vi "HORNSCAN_PERFORMANCE_40KHZ.vi"() -> ()   [LabVIEW 2017]
panel:
  out "Test Result":picture
  out "XY Graph":cluster{dbl, u32}[](graph)
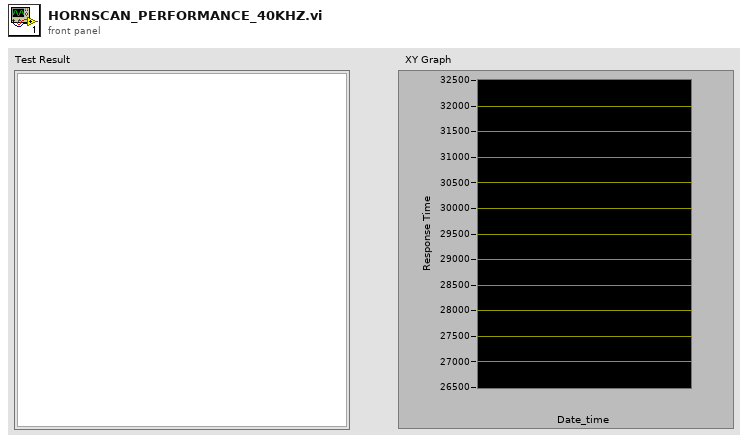
[diagram p1: front panel]
types:
  T1 = enum16{"open", "replace", "create", "open or create", "replace or create", "replace or create with confirmation"}
  T2 = cluster{"[0]":string, "[1]":string, "[2]":string, "[3]":string, "[4]":string, "[5]":string, "[6]":string, "[7]":string, "[8]":string}
  T3 = cluster{"Iterations":u64, "DelayBetweenIterations":u32, "Timeout":u32, "MessageID":i32, "MessageLength":i32, "ResponseID":i32, "Timestamp":string, "TestSuite":string, "ReportPath":path, "FWVersionPath":path}
  T4 = cluster{"Socket_IP_Address":string, "Socket_Port_Number":u16, "Global_ReportPath":path}
  T5 = typedef "imagedata.ctl" = cluster{"image type":i32, "image depth":i32, "image":u8[], "mask":u8[], "colors":u32[], "Rectangle":cluster{"left":i16, "top":i16, "right":i16, "bottom":i16}}
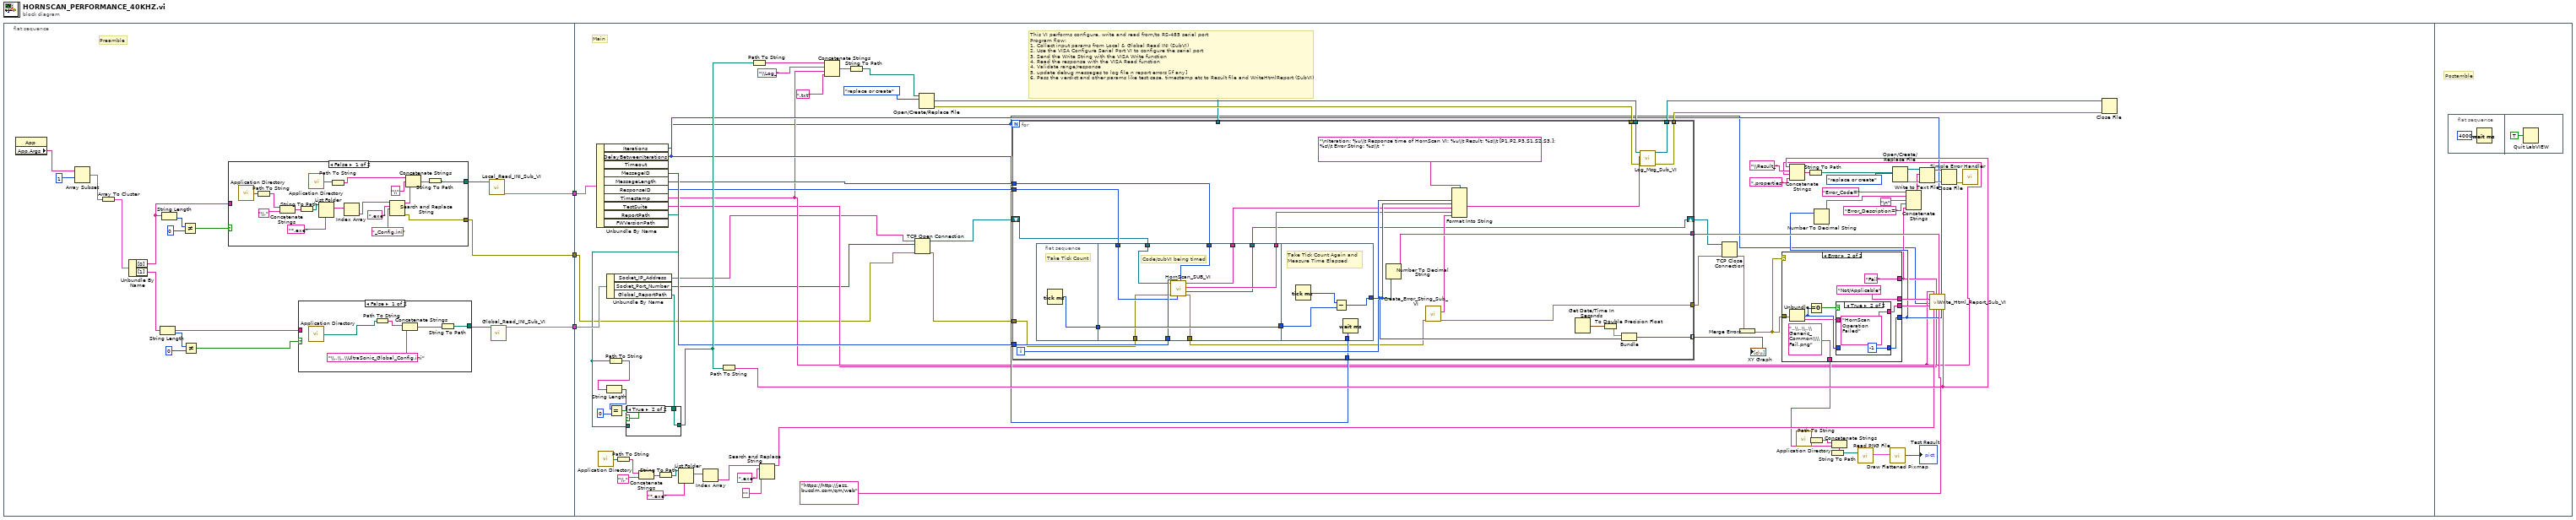
[diagram p0: block diagram]
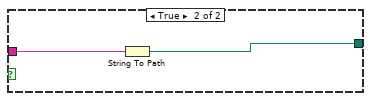
[diagram p2: hidden frame]
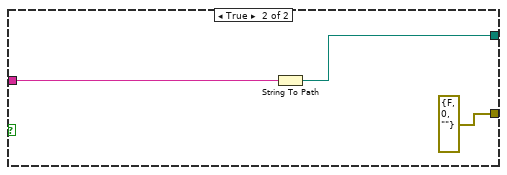
[diagram p3: hidden frame]
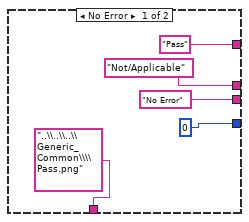
[diagram p5: hidden frame]
diagram:
  n1 = flat-sequence {
    tunnel: [w6] -> w3
    tunnel: [w5] -> w2
    tunnel: [w4] -> w1
    tunnel: w3 -> [w55]
    tunnel: w2 -> [w67]
    tunnel: w1 -> [w65]
    frame #0 {
      # "Preamble"
      n2 = property class="App"() -> ("App.Args"=w8:string[])  [unwired: 2 in, 2 out]
      n3 = Array Subset "Array Subset"(array=w8, index=1) -> (w9:string[])  [unwired: 1 in]
      n4 = Array To Cluster(array=w9) -> (cluster=w10:T2)
      n5 = Unbundle By Name "Unbundle By Name"(w10) -> ("[0]"=w14:string, "[1]"=w17:string)
      n6 = String Length(string=w17) -> (length=w18:i32)
      n7 = String Length(string=w14) -> (length=w11:i32)
      n8 = Not Equal?(x=w11, y=0) -> (x != y?=w13:bool)
      n9 = Not Equal?(x=w18, y=0) -> (x != y?=w16:bool)
      n10 = case shown="False" w13 {
        tunnel: w14 -> [_ w47]
        tunnel: [w29 w46] -> w19
        tunnel: [w28 errorcluster {"status"=FALSE, "code"=0, "source"=""} ("error out")] -> w6
        frame False {
          n11 = call <vilib>:"Application Directory.vi"() -> ("Application Directory"=w35:path)
          n12 = Path To String(path=w35) -> (string=w34:string)
          n13 = Concatenate Strings(w34, "\\." ("string")) -> (w32:string)
          n14 = String To Path(string=w32) -> (path=w37:path)
          n15 = call <vilib>:"Application Directory.vi"() -> ("Application Directory"=w44:path)
          n16 = List Folder(path=w37, pattern="*.exe") -> (filenames=w31:string[])  [unwired: 2 in, 3 out]
          n17 = Path To String(path=w44) -> (string=w39:string)
          n18 = Index Array(array=w31) -> (element=w30:string)  [unwired: 1 in]
          n19 = Search and Replace String(input string=w30, search string=".exe", replace string="_Config.ini" ("replace string (\"\")")) -> (result string=w41:string, error out=w28:errorcluster)  [unwired: 5 in, 2 out]
          n20 = Concatenate Strings(w39, "\\" ("string"), w41) -> (w38:string)
          n21 = String To Path(string=w38) -> (path=w29:path)
        }
        frame True {
          n22 = String To Path(string=w47) -> (path=w46:path)
        }
      }
      n23 = case shown="False" w16 {
        tunnel: [w22 w27] -> w20
        tunnel: w17 -> [_ w26]
        frame False {
          n24 = call <vilib>:"Application Directory.vi"() -> ("Application Directory"=w21:path)
          n25 = Path To String(path=w21) -> (string=w25:string)
          n26 = Concatenate Strings(w25, "\\..\\..\\UltraSonic_Global_Config.ini" ("string")) -> (w23:string)
          n27 = String To Path(string=w23) -> (path=w22:path)
        }
        frame True {
          n28 = String To Path(string=w26) -> (path=w27:path)
        }
      }
      n29 = call "Local_Read_INI_Sub_VI.vi"("Config File Path"=w19) -> ("output cluster"=w4:T3)  [unwired: 10 in]
      n30 = call "Global_Read_INI_Sub_VI.vi"("Config File Path"=w20) -> ("output cluster"=w5:T4)  [unwired: 14 in]
    }
    frame #1 {
      # "This VI performs configure, write and read from/to RS-485 serial port\nProgram flow:\n1. Collect input params from Local & Global Read INI (SubVI)\n2. Use the VISA Configure Serial Port VI to configure the serial port\n3. Send the Write String with the VISA Write function\n4. Read the response with the VISA Read function\n4. Validate range/response\n5. update debug messages to log file n report errors [if any]\n6. Pass the verdict and other params like test case, timestamp etc to Result file and WriteHtmlReport (SubVI)"
      # "Main"
      n31 = Unbundle By Name(w65) -> ("Iterations"=w57:u64, "DelayBetweenIterations"=w61:u32, "MessageID"=w64:i32, "MessageLength"=w63:i32, "ResponseID"=w62:i32, "Timestamp"=w59:string, "TestSuite"=w58:string, "ReportPath"=w56:path)  [unwired: 2 out]
      n32 = call <vilib>:"Application Directory.vi"() -> ("Application Directory"=w83:path)
      n33 = Unbundle By Name(w67) -> ("Socket_IP_Address"=w48:string, "Socket_Port_Number"=w52:u16, "Global_ReportPath"=w66:path)
      n34 = Path To String(path=w56) -> (string=w113:string)
      n35 = String Length(string=w113) -> (length=w112:i32)
      n36 = Equal?(x=w112, y=0) -> (x = y?=w110:bool)
      n37 = Path To String(path=w83) -> (string=w82:string)
      n38 = case shown="True" w110 {
        tunnel: w66 -> [_ w125]
        tunnel: [w124 w125] -> w109
        tunnel: w56 -> [w124 _]
        frame False {
        }
        frame True {
        }
      }
      n39 = Concatenate Strings(w82, "\\." ("string")) -> (w80:string)
      n40 = String To Path(string=w80) -> (path=w85:path)
      n41 = List Folder(path=w85, pattern="*.exe") -> (filenames=w79:string[])  [unwired: 2 in, 3 out]
      n42 = Index Array(array=w79) -> (element=w75:string)  [unwired: 1 in]
      n43 = Path To String(path=w109) -> (string=w86:string)
      n44 = Path To String(path=w109) -> (string=w115:string)
      n45 = Search and Replace String(input string=w75, search string=".exe", replace string="" ("replace string (\"\")")) -> (result string=w78:string)  [unwired: 5 in, 3 out]
      n46 = Concatenate Strings(w115, "\\Log_" ("string"), w59, ".txt" ("string")) -> (w118:string)
      n47 = String To Path(string=w118) -> (path=w117:path)
      n48 = TCP Open Connection(address=w48, remote port or service name=w52, error in (no error)=w55) -> (connection ID=w53:refnum<k5>, error out=w54:errorcluster)  [unwired: 2 in]
      n49 = Open/Create/Replace File(file path (use dialog)=w117, operation (0:open)=T1."replace or create") -> (refnum out=w87:refnum<file>, error out=w90:errorcluster)  [unwired: 1 in, 4 out]
      n50 = for {
        N: w57 -> [_]
        tunnel: [w149] -> w121
        tunnel: w87 -> [w143]
        tunnel: [w142] -> w89
        tunnel: [w140] -> w88
        tunnel: [w145] -> w119 mode=indexing
        tunnel: w90 -> [w141]
        tunnel: w87 -> [_]
        tunnel: [w137] -> w51
        tunnel: w64 -> [w136]
        tunnel: w63 -> [w135]
        tunnel: w62 -> [w131]
        tunnel: w61 -> [w133]
        tunnel: w54 -> [w130]
        shift-right: [w126] -> w49
        shift-left: w53 -> [w127]
        i -> [w138]
        n51 = flat-sequence {
          tunnel: [w152] -> w151
          tunnel: [w162] -> w150
          tunnel: w151 -> [w162]
          tunnel: w136 -> [w160]
          tunnel: w135 -> [w158]
          tunnel: w131 -> [w159]
          tunnel: [w161] -> w134
          tunnel: [w156] -> w132
          tunnel: w130 -> [w157]
          tunnel: [w155] -> w128
          tunnel: w127 -> [w154]
          tunnel: [w153] -> w126
          tunnel: w150 -> [w166]
          tunnel: [w164] -> w139
          tunnel: w133 -> [w163]
          frame #0 {
            # "Take Tick Count"
            n52 = Tick Count (ms)() -> (millisecond timer value=w152:u32)
          }
          frame #1 {
            # "Code/subVI being timed"
            n53 = call "HornScan_SUB_VI.vi"("MessageLength"=w158, "Response ID"=w159, "Message ID"=w160, "error in (no error)"=w157, "connection ID"=w154) -> ("error out"=w156:errorcluster, "connection ID_out"=w153:refnum<k5>, "Resonant Frequencies"=w155:string, "Pass"=w161:string)  [unwired: 2 in]
          }
          frame #2 {
            # "Take Tick Count Again and Measure Time Elapsed"
            n54 = Tick Count (ms)() -> (millisecond timer value=w165:u32)
            n55 = Subtract(x=w165, y=w166) -> (x-y=w164:u32)
            n56 = Wait (ms)(milliseconds to wait=w163) -> ()  [unwired: 1 out]
          }
        }
        n57 = Number To Decimal String(number=w139) -> (decimal integer string=w149:string)  [unwired: 1 in]
        n58 = call "Create_Error_String_Sub_VI.vi"("error in"=w132) -> ("error out"=w137:errorcluster, "Error String"=w129:string)  [unwired: 9 in]
        n59 = Format Into String(format string="\nIteration: %u\\t Response time of HornScan VI: %u\\t Result: %s\\t [P1,P2,P3,S1,S2,S3,]: %s\\t Error String: %s\\t  ", w138, w139, w134, w128, w129) -> (resulting string=w144:string)  [unwired: 2 in, 1 out]
        n60 = Get Date/Time In Seconds() -> (seconds since 1Jan1904=w146:timestamp)
        n61 = To Double Precision Float(number=w146) -> (double precision float=w147:dbl)
        n62 = Bundle "Bundle"(w147, w139) -> (w145:cluster{dbl, u32})  [unwired: 1 in]
        n63 = call "Log_Msg_Sub_VI.vi"("error in (no error)"=w141, "String"=w144, "Byte Stream File in"=w143) -> ("error out"=w140:errorcluster, "Byte Stream File out"=w142:refnum<file>)  [unwired: 7 in]
      }
      "XY Graph" <- w119
      n64 = TCP Close Connection(connection ID=w49, error in (no error)=w51) -> (error out=w50:errorcluster)  [unwired: 1 in, 1 out]
      n65 = Merge Errors "Merge Errors"(w50) -> (w60:errorcluster)
      n66 = case shown="Error" w60 {
        tunnel: ["Pass" "Fail"] -> w91
        tunnel: w60 -> [_ w178]
        tunnel: [0 ("code") w174] -> w95
        tunnel: ["No Error" ("source") w175] -> w123
        tunnel: ["Not/Applicable" "Not/Applicable"] -> w122
        tunnel: ["..\\..\\..\\Generic_Common\\\\Pass.png" ("string") "..\\..\\..\\Generic_Common\\\\Fail.png" ("string")] -> w68
        frame No Error {
        }
        frame Error {
          n67 = Unbundle(w178) -> ("code"=w176:i32, "source"=w172:string)  [unwired: 1 out]
          n68 = Equal To 0?(x=w176) -> (x = 0?=w173:bool)
          n69 = case shown="True" w173 {
            tunnel: [w182 -1 ("code")] -> w174
            tunnel: [w181 "HornScan Operation Failed" ("source")] -> w175
            tunnel: w176 -> [w182 _]
            tunnel: w172 -> [w181 _]
            frame False {
            }
            frame True {
            }
          }
        }
      }
      n70 = Concatenate Strings(w86, "\\Result_" ("string"), w59, ".properties" ("string")) -> (w107:string)
      n71 = call <vilib>:"Application Directory.vi"() -> ("Application Directory"=w69:path)
      n72 = String To Path(string=w107) -> (path=w99:path)
      n73 = Path To String(path=w69) -> (string=w70:string)
      n74 = Number To Decimal String(number=w95) -> (decimal integer string=w94:string)  [unwired: 1 in]
      n75 = Concatenate Strings(w70, w68) -> (w71:string)
      n76 = String To Path(string=w71) -> (path=w74:path)
      n77 = call <vilib>:"Read PNG File.vi"("path to PNG file"=w74) -> ("image data"=w72:T5)  [unwired: 8 in, 2 out]
      n78 = call <vilib>:"Draw Flattened Pixmap.vi"("image data"=w72) -> ("new picture"=→"Test Result":picture)  [unwired: 8 in]
      n79 = Open/Create/Replace File(file path (use dialog)=w99, operation (0:open)=T1."replace or create") -> (refnum out=w98:refnum<file>, error out=w103:errorcluster)  [unwired: 4 in, 1 out]
      n80 = Concatenate Strings("Error_Code=" ("string"), w94, "\n", "Error_Description=" ("string"), w91) -> (w97:string)
      n81 = Write to Text File(file (use dialog)=w98, text=w97, error in=w103) -> (refnum out=w102:refnum<file>, error out=w101:errorcluster)  [unwired: 1 in, 1 out]
      n82 = call "Write_Html_Report_Sub_VI.vi"("ReprtPath"=w86, "Remarks"=w122, "Iterations"=w57, "Error Description"=w123, "Timestamp"=w59, "TestCase"=w78, "Verdict"=w91, "TestSuite"=w58, "Time taken to execute  test in msec"=w121, "JazzDashboardLink"="https://http://jazz.bucclm.com/qm/web" ("TestSuite"), "Delay Between Iterations"=w61, "Error Code"=w95) -> ()  [unwired: 8 in]
      n83 = Close File(refnum=w102, error in=w101) -> (error out=w100:errorcluster)  [unwired: 1 out]
      n84 = call <vilib>:"Simple Error Handler.vi"("error in (no error)"=w100) -> ()  [unwired: 4 in, 5 out]
      n85 = Close File(refnum=w89, error in=w88) -> ()  [unwired: 2 out]
    }
    frame #2 {
      # "Postamble"
      n86 = flat-sequence {
        frame #0 {
          n87 = Wait (ms)(milliseconds to wait=u32 4000) -> ()  [unwired: 1 out]
        }
        frame #1 {
          n88 = Quit LabVIEW(quit? (T)=TRUE) -> ()
        }
      }
    }
  }
